vi "DAQmx task create-Pockels modulation AO.vi"(9 "Setup/Logging queue element":T1={"Imaging Protocol"=enum."Live Imaging", "Number of Trials"=0, "Frame Size"=512, "# Averaged frames"=0, "Dwell time (us)"=0.0, "Index of Z-plane"=0, "Timelapse?"=FALSE, "Logging process is active"=FALSE, "Speed logging enabled"=FALSE, "tdms file ref"=refnum, "path"=path "", "Trial Number"=0, "Expected # points acquired"=FALSE, "Manually stopped"=FALSE, "Last trial"=FALSE, "Ch0 data"=[], "Ch1 data"=[], "Ref Data"=[], "Ref Frame Time"=[], "Image Time"=[], "Continuous Time"=[], "Ref X Length"=0, "Ref Y Length"=0, "# Ref Averaged frames"=0, "Ref Dwell time (us)"=0.0, "Points acquired"={"Ch0 last trial"=0, "Ch1 last trial"=0, "All trials"=0}, "HW Timings File"=refnum} {"Ref Dwell time (us)" format="%#.6g"; "Frame Size" items=["100X100"=100, "128X128"=128, "200X200"=200, "256X256"=256, "512X512"=512, "1024x1024"=1024, "2048x2048"=2048]; "Dwell time (us)" format="%#.6g"}, 11 "Internal O/P reference of the \ncounter used as the AO clock":tag) -> (1 "error out":errorcluster, 2 "Data length (points)":i32, 3 "Pockels modulation AO task":refnum<k21>, 5 "Info":T5, 7 "Pockels modulation data out":dbl[](array[numeric]))   [LabVIEW 2020]
uses:
  Typedefs/Logging queue element.ctl
  Typedefs/Imaging Protocols enum.ctl
  Typedefs/Frame Size.ctl
  Typedefs/Acquired points count.ctl
  Typedefs/Functional Global Default States.ctl
  Typedefs/HW config states enum.ctl
  <vilib>/DAQmx/write.llb/DAQmx Write (Analog 1D DBL 1Chan NSamp).vi
  Globals/gl_Pockels control globals.vi
  <vilib>/DAQmx/create/channels.llb/DAQmx Create Channel (AO-Voltage-Basic).vi
  Global Variables/General Globals.vi
  <vilib>/DAQmx/configure/timing.llb/DAQmx Timing (Sample Clock).vi
  <vilib>/DAQmx/miscellaneous.llb/DAQmx Fill In Error Info.vi
  <resource>/objmgr/daqmx.rc
panel:
  out "Pockels control AO channel":tag="PXI1Slot4/ao0"
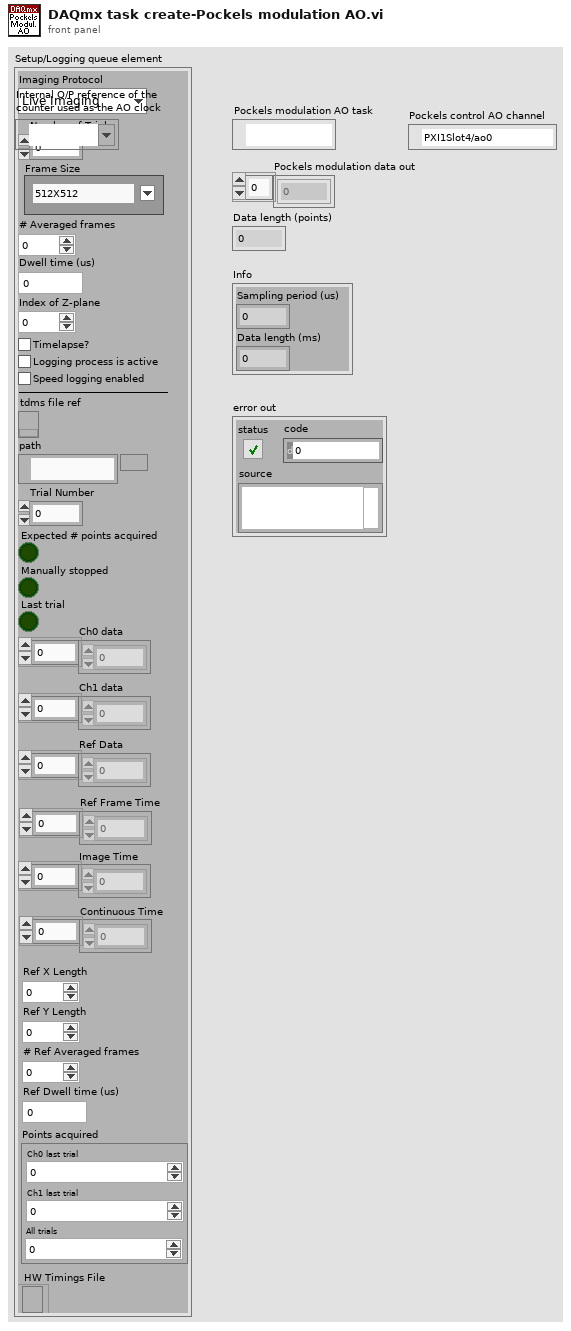
[diagram p1: front panel]
types:
  T1 = typedef "Logging queue element.ctl" = cluster{"Imaging Protocol":T2, "Number of Trials":u16, "Frame Size":T3, "# Averaged frames":u16, "Dwell time (us)":dbl, "Index of Z-plane":i32, "Timelapse?":bool, "Logging process is active":bool, "Speed logging enabled":bool, "tdms file ref":refnum<k34>, "path":path, "Trial Number":i32, "Expected # points acquired":bool, "Manually stopped":bool, "Last trial":bool, "Ch0 data":u32[], "Ch1 data":u32[], "Ref Data":u32[], "Ref Frame Time":u64[], "Image Time":u64[], "Continuous Time":u64[], "Ref X Length":u16, "Ref Y Length":u16, "# Ref Averaged frames":u16, "Ref Dwell time (us)":dbl, "Points acquired":T4, "HW Timings File":refnum<file>}
  T2 = typedef "Imaging Protocols enum.ctl" = enum16{"AOL Z-Stack", "Motor Z Stack", "Functional Acquisition", "Single Plane Acquisition", "Volume Acquisition", "Live Imaging", "Live Plane Imaging", "Live Volume Imaging"}
  T3 = typedef "Frame Size.ctl" = u16
  T4 = typedef "Acquired points count.ctl" = cluster{"Ch0 last trial":u64, "Ch1 last trial":u64, "All trials":u64}
  T5 = cluster{"Sampling period (us)":dbl, "Data length (ms)":dbl}
  T6 = cluster{"Sampling period (sec)":dbl, "Data length (us)":dbl}
  T7 = typedef "HW config states enum.ctl" = enum16{"Load from file", "Save to file", "Save backup", "Write all", "Read all", "Write XY stage settings", "Write DAQ FPGA settings", "Write Control FPGA settings", "Write Phys Channels", "Write System Config", "Write HW Config", "Save System Config", "Save HW Config", "Clear", "Compare from file"}
  T8 = typedef "Functional Global Default States.ctl" = enum16{"Read", "Write", "Clear"}
  T9 = typedef "Hardware Configuration settings.ctl" = cluster{"Dev. PC":bool, "Swap XY on stage":bool, "No of AOD":u8, "MC Supported":bool, "Axial MC":bool, "Computer MAC address":string, "Externalise Triggers":bool, "Trigger HW config":T10, "DAQmx Chan":T11, "XY stage available":bool, "XY Stage":T12, "Z stage available":bool, "Z Stage config cluster":T13, "Encoder available":bool, "Encoder":T14, "VidRec available":bool, "Cam VidRec":T15, "Laser Power Control HW config":T16, "Laser 1 available":bool, "Laser 1 config cluster":T17, "Prechirper 1 available":bool, "Prechirper 1 config cluster":T18, "Control system.FPGA available?":bool, "Control Sys. HW config":T19, "DAQ FPGA HW Config":T20, "PMT Voltage Range":T24}
  T10 = typedef "Triggers HW config.ctl" = cluster{"Available Device List":i32, "Device Address":string}
  T11 = typedef "DAQmx physical channels cluster.ctl" = cluster{"Pockels AO":tag, "Hard shutter AO":tag, "PMT AOs":tag, "Galvo AOs":tag, "Power meter AI":tag}
  T12 = typedef "XY Stage config cluster.ctl" = cluster{"COM port":refnum<visa-resource-name>, "Baudrate":i32, "Type":string}
  T13 = typedef "Z Stage config cluster.ctl" = cluster{"COM port":refnum<visa-resource-name>, "Baudrate":i32, "Type":string}
  T14 = typedef "Encoder config cluster.ctl" = cluster{"IP address":string, "Port":u16, "Wheel radius (cm)":dbl, "Encoder Trigger":tag}
  T15 = typedef "Cam VidRec HW config setup cluster.ctl" = cluster{"DO flag-Video record":tag, "DO flag-Trial start":tag}
  T16 = typedef "Laser Power Control HW config.ctl" = cluster{"Laser Power Control":string, "Laser Power Modulation Control":enum16{"NI", "FPGA"}}
  T17 = typedef "Laser 1 config cluster.ctl" = cluster{"COM port":refnum<visa-resource-name>, "Baud Rate":i32, "Type":string}
  T18 = typedef "PreChirper 1 config cluster.ctl" = cluster{"Type":string, "Baud Rate":i32, "COM port":refnum<visa-resource-name>}
  T19 = typedef "Control Sys HW config cluster.ctl" = cluster{"Control system.FPGA Type":enum16{"Virtex 5", "Virtex 7"}, "Control system.Network adapter name":string, "Control system.MAC address":string, "Control system.Ethernet Port":u32, "Control system.Ethernet Port Opened":bool}
  T20 = typedef "DAQ FPGA HW config cluster.ctl" = cluster{"FGPA Ref":T21, "Target":T22, "input card type":T23}
  T21 = typedef "FPGA Ref.ctl" = refnum<k20>
  T22 = typedef "nirio_resource_hc.ctl" = tag
  T23 = typedef "FPGA input type AC-DC.ctl" = enum16{"AC Card", "DC Card"}
  T24 = typedef "PMT Voltage Range.ctl" = cluster{"PMT Voltage Lower Limit":dbl, "PMT Voltage Upper Limit":dbl}
  T25 = cluster{"Sampling period (us)":dbl, "Length of sequence (ms)":dbl}
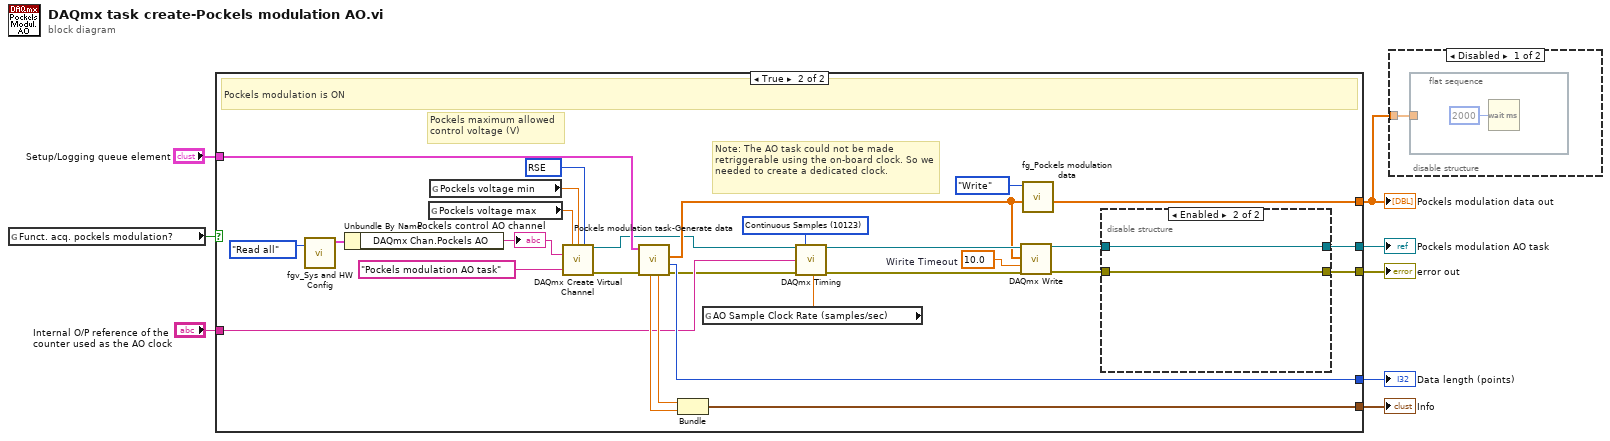
[diagram p0: block diagram]
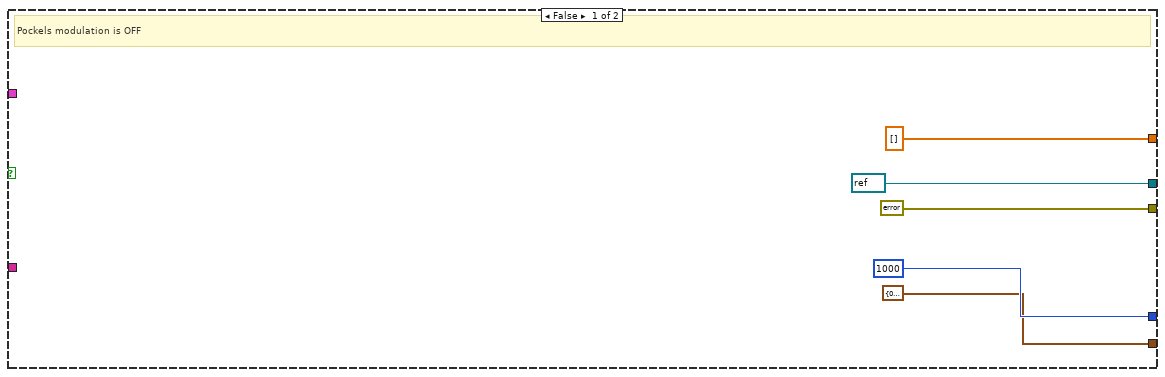
[diagram p3: hidden frame]
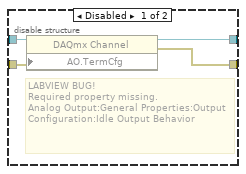
[diagram p4: hidden frame]
diagram:
  n1 = global read "gl_Pockels control globals.vi" "Funct. acq. pockels modulation?"() -> (w3:bool)
  n2 = case shown="True" w3 {
    tunnel: [errorcluster {"status"=FALSE, "code"=0, "source"=""} ("error out") w19] -> w5
    tunnel: [refnum<k21> refnum ("task out") w21] -> w6
    tunnel: [1000 ("Number of samples in AO sequence") w39] -> w4
    tunnel: "Setup/Logging queue element" -> [_ w38]
    tunnel: [T6 {"Sampling period (sec)"=0.0, "Data length (us)"=0.0} w37] -> w8
    tunnel: "Internal O/P reference of the \ncounter used as the AO clock" -> [_ w34]
    tunnel: [dbl[] [] ("Pockels modulation data out") w26] -> w1
    frame False {
      # "Pockels modulation is OFF"
    }
    frame True {
      w18 = 10083 items=["Default"=-1, "RSE"=10083, "Differential"=10106, "Pseudodifferential"=12529] ("output terminal configuration")
      w29 = 10.0  # Wirite Timeout
      w28 = 10123 items=["Finite Samples"=10178, "Continuous Samples"=10123] ("sample mode")
      # "Note: The AO task could not be made retriggerable using the on-board clock. So we needed to create a dedicated clock."
      # "Pockels maximum allowed control voltage (V)"
      # "Pockels modulation is ON"
      n3 = call "fgv_Sys and HW Config.vi"("Function"=HW_config_states_enum."Read all") -> ("Hardware Configuration OUT"=w15:T9)  [unwired: 8 in, 2 out]
      n4 = Unbundle By Name(w15) -> ("DAQmx Chan.Pockels AO"=w14:tag)
      "Pockels control AO channel" <- w14
      n5 = global read "gl_Pockels control globals.vi" "Pockels voltage max"() -> (w24:dbl)
      n6 = global read "gl_Pockels control globals.vi" "Pockels voltage min"() -> (w23:dbl)
      n7 = call-poly <vilib>:"DAQmx Create Virtual Channel.vi"("maximum value"=w24, "minimum value"=w23, "output terminal configuration"=w18, "physical channels"=w14, "name to assign"="Pockels modulation AO task") -> ("task out"=w22:refnum<k21>, "error out"=w40:errorcluster)  [unwired: 9 in]
      n8 = call "Pockels modulation task-Generate data.vi"("error in (no error)"=w40, "Setup/Logging queue element"=w38) -> ("error"=w32:errorcluster, "Data length (points)"=w39:i32, "Pockels modulation data"=w25:dbl[], "Sampling period (us)"=w36:dbl, "Length of sequence (ms)"=w35:dbl)  [unwired: 5 in]
      n9 = Bundle("Sampling period (us)"=w36, "Length of sequence (ms)"=w35) -> (w37:T25)  [unwired: 1 in]
      n10 = global read "General Globals.vi" "AO Sample Clock Rate (samples/sec)"() -> (w17:dbl)
      n11 = call-poly <vilib>:"DAQmx Timing.vi"("task/channels in"=w22, "sample mode"=w28, "rate"=w17, "source"=w34, "error in"=w32) -> ("task out"=w30:refnum<k21>, "error out"=w31:errorcluster)  [unwired: 9 in]
      n12 = call-poly <vilib>:"DAQmx Write.vi"("task/channels in"=w30, "data"=w25, "timeout"=w29, "error in"=w31) -> ("task out"=w33:refnum<k21>, "error out"=w20:errorcluster)  [unwired: 9 in, 1 out]
      n13 = call "fg_Pockels modulation data.vi"("Pockels modulation data in"=w25, "Function"=Functional_Global_Default_States."Write") -> ("Pockels modulation data out"=w26:dbl[])  [unwired: 9 in]
      n14 = disable-structure shown="Enabled" {
        disable-tunnel: w33 -> [w45 w47]
        disable-tunnel: [w44 w47] -> w21
        disable-tunnel: w20 -> [w43 w46]
        disable-tunnel: [w42 w46] -> w19
        frame Disabled {
          # "LABVIEW BUG!\nRequired property missing.\nAnalog Output:General Properties:Output Configuration:Idle Output Behavior"
          n15 = property class="DAQmx Channel" props=["AO.TermCfg"](reference=w45, error in=w43) -> (reference out=w44:refnum<k21>, error out=w42:errorcluster)  [unwired: 1 in]
        }
        frame Enabled {
        }
      }
    }
  }
  "Info" <- w8
  "Pockels modulation data out" <- w1
  "Data length (points)" <- w4
  "error out" <- w5
  "Pockels modulation AO task" <- w6
  n16 = disable-structure shown="Disabled" {
    disable-tunnel: w1 -> [w48 _]
    frame Disabled {
      n17 = flat-sequence {
        tunnel: w48 -> [_]
        frame #0 {
          n18 = Wait (ms)(milliseconds to wait=u32 2000) -> ()  [unwired: 1 out]
        }
      }
    }
    frame Enabled {
    }
  }
